vi "TDMS Advanced Ring Buffer.vi"() -> ()   [LabVIEW 2023]
doc: "This example demonstrates how to overwrite data repeatedly from a specified position in an existing .tdms file using the Advanced TDMS VIs and functions, to view the pre-triggered data in a ring buffer use case."
uses:
  <vilib>/Analysis/NI_AALBase.lvlib
panel:
  out "Write Buffer Status":dbl(graph)
  out "XY Graph":cluster{dbl[], dbl[]}[](graph)
  in  "Trigger":bool
  in  "Pre-Trigger [number of samples]":i32=100
  in  "Number of Samples":i32=12800
  # "Overview: Demonstrates the use of the Advanced TDMS functions to overwrite data repeatedly from a specified position in an existing .tdms file, to view the pre-triggered data in a ring buffer use case.\nInstructions:\n1. Run this VI.\n2. Click the Trigger button and view the pre-triggered data in a ring buffer use case.\n3. Delete the .tdms file (located at [LabVIEW Data]\\Example TDMS Advanced Ring Buffer.tdms) when you are done."
  # "Data Acquisition (simulated)"
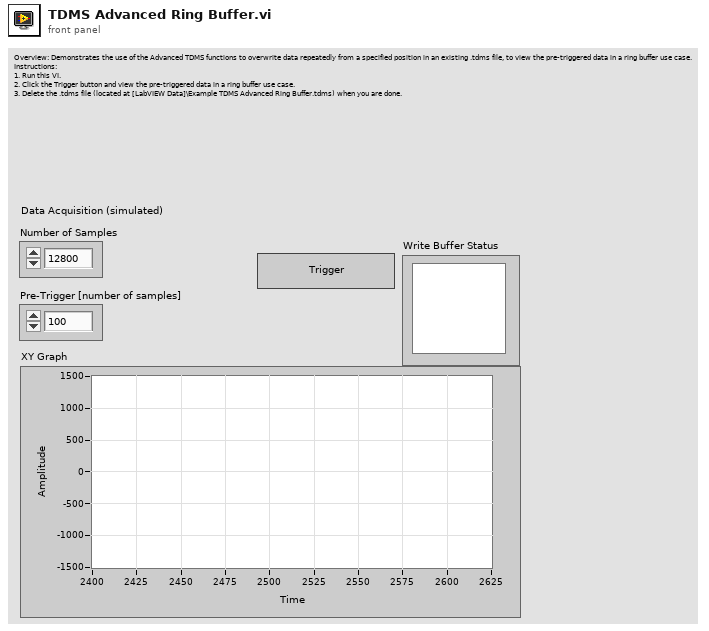
[diagram p1: front panel]
types:
  T1 = enum16{"open", "open or create", "create or replace", "create", "open (read-only)"}
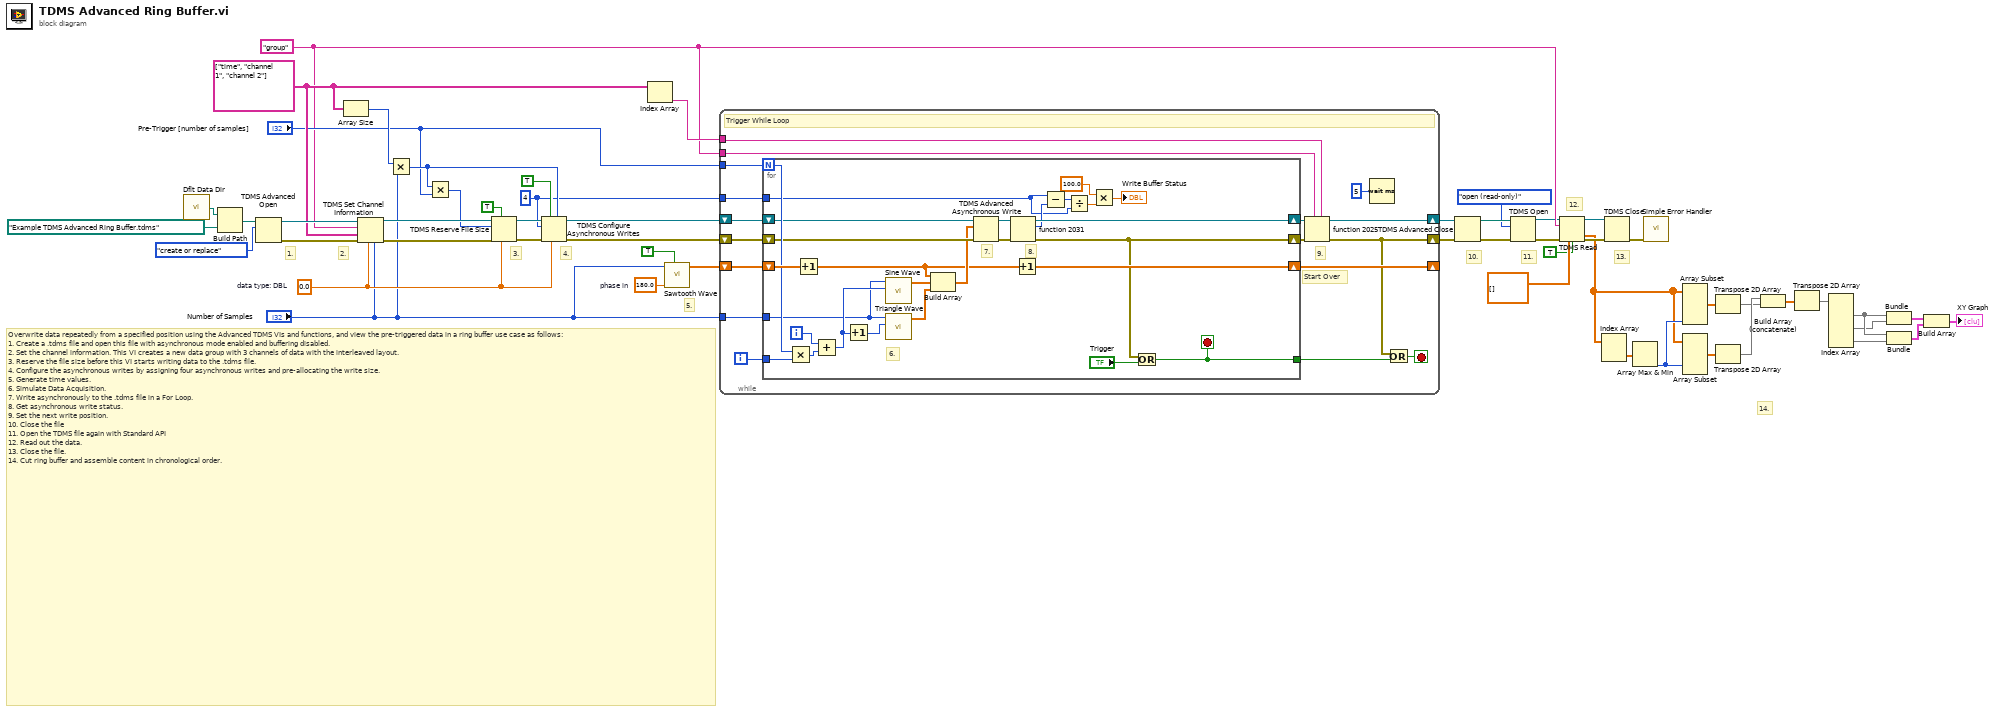
[diagram p0: block diagram]
diagram:
  w38 = 180.0  # phase in
  w8 = u32 4 ("number of buffers (4)")
  w44 = 0.0  # data type: DBL
  w35 = string[] ["time", "channel 1", "channel 2"] ("channel name(s)")
  w25 = "group" ("group name (Untitled)")
  # "Overwrite data repeatedly from a specified position using the Advanced TDMS VIs and functions, and view the pre-triggered data in a ring buffer use case as follows:\n1. Create a .tdms file and open this file with asynchronous mode enabled and buffering disabled.\n2. Set the channel information. This VI creates a new data group with 3 channels of data with the interleaved layout. \n3. Reserve the file size before this VI starts writing data to the .tdms file. \n4. Configure the asynchronous writes by assigning four asynchronous writes and pre-allocating the write size.\n5. Generate time values.\n6. Simulate Data Acquisition.\n7. Write asynchronously to the .tdms file in a For Loop.\n8. Get asynchronous write status.\n9. Set the next write position.\n10. Close the file\n11. Open the TDMS file again with Standard API\n12. Read out the data.\n13. Close the file.\n14. Cut ring buffer and assemble content in chronological order."
  # "13."
  # "12."
  # "11."
  # "10."
  # "14."
  # "5."
  # "4."
  # "1."
  # "3."
  # "2."
  n1 = call <vilib>:"Dflt Data Dir.vi"() -> ("App:Default Data Directory"=w49:path)
  n2 = Build Path(base path=w49, name or relative path=path "Example TDMS Advanced Ring Buffer.tdms") -> (appended path=w53:path)
  n3 = TDMS Advanced Open(10:T1."create or replace" ("operation (0:open)"), 11:w53) -> (0:w51:errorcluster, 3:w50:refnum<k34>)  [unwired: 3 in, 1 out]
  n4 = Array Size(array=w35) -> (size(s)=w34:i32)
  n5 = TDMS Set Channel Information(4:"Number of Samples", 6:w44, 8:w51, 9:w35, 10:w25, 11:w50) -> (0:w48:errorcluster, 3:w47:refnum<k34>)  [unwired: 1 in]
  n6 = Multiply(x=w34, y="Number of Samples") -> (x*y=w33:i32)
  n7 = Multiply(x=w33, y="Pre-Trigger [number of samples]") -> (x*y=w31:i32)
  n8 = TDMS Reserve File Size(6:w44, 7:TRUE ("append? (T)"), 8:w48, 10:w31, 11:w47) -> (0:w46:errorcluster, 3:w45:refnum<k34>)
  n9 = TDMS Configure Asynchronous Writes(5:w33, 6:w44, 7:TRUE ("pre-allocate? (F)"), 8:w46, 10:w8, 11:w45) -> (0:w6:errorcluster, 3:w39:refnum<k34>)  [unwired: 1 in]
  n10 = Index Array(array=w35) -> (element=w40:string)  [unwired: 1 in]
  n11 = call <vilib>:"Sawtooth Wave.vi"("samples"="Number of Samples", "phase in"=w38, "reset phase"=TRUE) -> ("sawtooth wave"=w37:dbl[])  [unwired: 2 in, 2 out]
  n12 = while {
    tunnel: w25 -> [w71]
    tunnel: w40 -> [w70]
    shift-right: [w61] -> w41
    shift-left: w39 -> [w69]
    shift-right: [w55] -> w42
    shift-left: w6 -> [w68]
    shift-right: [w64] -> _
    shift-left: w37 -> [w65]
    tunnel: "Number of Samples" -> [w62]
    tunnel: "Pre-Trigger [number of samples]" -> [w60]
    tunnel: w8 -> [w57]
    i -> [w63]
    stop <- w59 stop-if-true
    # "9."
    # "Start Over"
    # "Trigger While Loop"
    n13 = for {
      N: w60 -> [w97]
      shift-right: [w79] -> w66
      shift-left: w69 -> [w92]
      shift-right: [w72] -> w67
      shift-left: w68 -> [w91]
      shift-right: [w83] -> w64
      shift-left: w65 -> [w98]
      tunnel: w63 -> [w96]
      tunnel: w62 -> [w86]
      tunnel: [w87] -> w58
      tunnel: w57 -> [w76]
      i -> [w94]
      stop <- w87 stop-if-true
      # "8."
      # "7."
      # "6."
      n14 = Multiply(x=w97, y=w96) -> (x*y=w95:i32)
      n15 = Increment(x=w98) -> (x+1=w82:dbl[])
      n16 = Add(x=w94, y=w95) -> (x+y=w93:i32)
      n17 = Increment(x=w93) -> (x+1=w85:i32)
      n18 = call <vilib>:"Sine Wave.vi"("samples"=w86, "amplitude"=w93) -> ("sine wave"=w90:dbl[])  [unwired: 3 in, 2 out]
      n19 = call <vilib>:"Triangle Wave.vi"("samples"=w86, "amplitude"=w85) -> ("triangle wave"=w84:dbl[])  [unwired: 3 in, 2 out]
      n20 = Build Array(w82, w90, w84) -> (w89:dbl[][])
      n21 = TDMS Advanced Asynchronous Write(8:w91, 10:w89, 11:w92) -> (0:w81:errorcluster, 3:w80:refnum<k34>)
      n22 = fn#2031(8:w81, 11:w80) -> (0:w72:errorcluster, 2:w78:u32, 3:w79:refnum<k34>)
      n23 = Increment(x=w82) -> (x+1=w83:dbl[])
      n24 = Subtract(x=w76, y=w78) -> (x-y=w77:u32)
      n25 = Divide(x=w77, y=w76) -> (x/y=w75:dbl)
      n26 = Multiply(x=100.0, y=w75) -> (x*y=→"Write Buffer Status":dbl)
      n27 = Or(x=w72, y="Trigger") -> (x .or. y?=w87:bool)
    }
    n28 = fn#2025(5:w70, 7:w71, 8:w67, 11:w66) -> (0:w55:errorcluster, 3:w61:refnum<k34>)  [unwired: 2 in]
    n29 = Wait (ms)(milliseconds to wait=u32 5) -> ()  [unwired: 1 out]
    n30 = Or(x=w55, y=w58) -> (x .or. y?=w59:bool)
  }
  n31 = TDMS Advanced Close(8:w42, 11:w41) -> (0:w26:errorcluster, 3:w28:path)  [unwired: 2 in]
  n32 = TDMS Open(8:w26, 10:T1."open (read-only)" ("operation (0:open)"), 11:w28) -> (0:w5:errorcluster, 3:w4:refnum<k34>)  [unwired: 4 in]
  n33 = TDMS Read(0:w4, 5:w25, 11:w5, 12:dbl[][] [] ("sawtooth wave"), 13:TRUE ("return channels in file order? (F)")) -> (4:w21:refnum<k34>, 10:w1:dbl[][], 15:w20:errorcluster)  [unwired: 3 in, 3 out]
  n34 = Index Array(array=w1) -> (element=w23:dbl[])  [unwired: 2 in]
  n35 = TDMS Close(8:w20, 11:w21) -> (0:w19:errorcluster)  [unwired: 1 out]
  n36 = Array Max & Min(array=w23) -> (min index (indices)=w22:i32)  [unwired: 3 out]
  n37 = call <vilib>:"Simple Error Handler.vi"("error in (no error)"=w19) -> ()  [unwired: 4 in, 5 out]
  n38 = Array Subset(array=w1, length (col)=w22) -> (w14:dbl[][])  [unwired: 3 in]
  n39 = Array Subset(array=w1, index (col)=w22) -> (w13:dbl[][])  [unwired: 3 in]
  n40 = Transpose 2D Array(2D array=w14) -> (transposed array=w10:dbl[][])
  n41 = Transpose 2D Array(2D array=w13) -> (transposed array=w11:dbl[][])
  n42 = Build Array (concatenate)(w11, w10) -> (w12:dbl[][])
  n43 = Transpose 2D Array(2D array=w12) -> (transposed array=w9:dbl[][])
  n44 = Index Array(array=w9) -> (element #1=w18:dbl[], element #2=w3:dbl[], element #3=w2:dbl[])  [unwired: 6 in]
  n45 = Bundle(w18, w3) -> (w16:cluster{dbl[], dbl[]})  [unwired: 1 in]
  n46 = Bundle(w18, w2) -> (w17:cluster{dbl[], dbl[]})  [unwired: 1 in]
  n47 = Build Array(w16, w17) -> (→"XY Graph":cluster{dbl[], dbl[]}[])
